vi "等分取数据.vi"(0 "Max":dbl, 1 "MIN":dbl, 3 "num":i32) -> (7 "数据点":dbl[](array[numeric]))   [LabVIEW 2010]
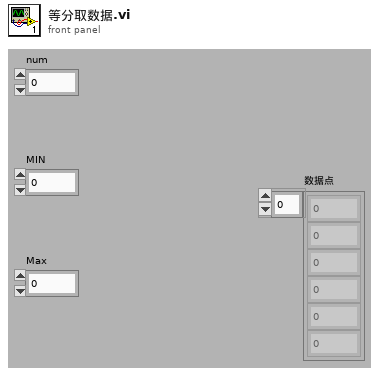
[diagram p1: front panel]
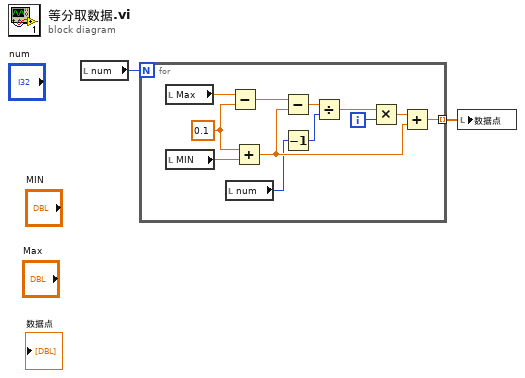
[diagram p0: block diagram]
diagram:
  n1 = local read "num"() -> (w1:i32)
  n2 = for {
    N: w1 -> [_]
    tunnel: [w11] -> w2 mode=indexing
    i -> [w10]
    w6 = 0.1
    n3 = local read "Max"() -> (w9:dbl)
    n4 = local read "MIN"() -> (w7:dbl)
    n5 = local read "num"() -> (w4:i32)
    n6 = Subtract(x=w9, y=w6) -> (x-y=w8:dbl)
    n7 = Add(x=w6, y=w7) -> (x+y=w5:dbl)
    n8 = Subtract(x=w8, y=w5) -> (x-y=w14:dbl)
    n9 = Decrement(x=w4) -> (x-1=w3:i32)
    n10 = Divide(x=w14, y=w3) -> (x/y=w13:dbl)
    n11 = Multiply(x=w13, y=w10) -> (x*y=w12:dbl)
    n12 = Add(x=w12, y=w5) -> (x+y=w11:dbl)
  }
  n13 = local write "数据点"(w2) -> ()
